vi "MUX_CommandsGlobal.vi"() -> ()   [LabVIEW 2013, in "Switching.lvclass"]
uses:
  Switching.lvclass
panel:
  in  "MUX GPIB Setup":T1={"Mux1 address"="", "Mux2 address"="", "Instrument name"="", "Instrument type"=2, "Command \"MUX Reset\""="", "Command \"Select MUX Channel\""=""} {"Instrument type" items=["Supply", "LCR", "Switching"]}
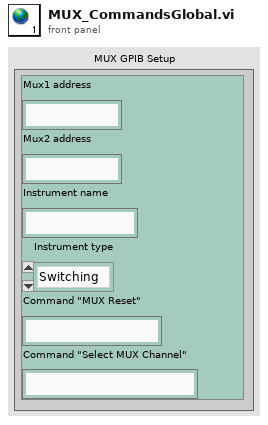
[diagram p1: front panel]
types:
  T1 = cluster{"Mux1 address":string, "Mux2 address":string, "Instrument name":string, "Instrument type":u16, "Command \"MUX Reset\"":string, "Command \"Select MUX Channel\"":string}
diagram:
